vi "Numeric Output Item Init.vi"(7 "Project In":refnum<class "Project.lvclass">, 8 "error in (no error)":errorcluster, 9 "Numeric UI Elements":T1, 10 "Output":T2, 11 "VI in":refnum<vi>) -> (0 "error out":errorcluster)   [LabVIEW 2015, in "OutputUI.lvclass"]
uses:
  OutputUI.lvclass
  Step/STEP_OUTPUT.ctl
  Step/OUTPUT_DATA_TYPE.ctl
  OUTPUT_CHECK_TYPE.ctl
  Step/OUTPUT_VALUE_TYPE.ctl
  Project.lvclass
  Step.lvclass
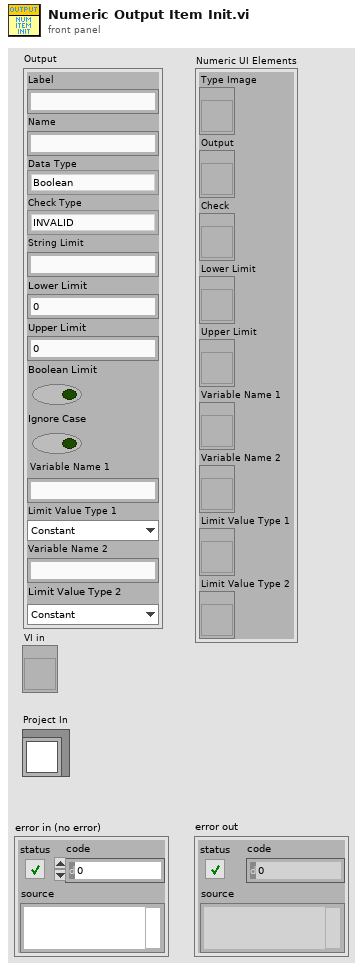
[diagram p1: front panel]
types:
  T1 = cluster{"Type Image":refnum<vi>, "Output":refnum<vi>, "Check":refnum<vi>, "Lower Limit":refnum<vi>, "Upper Limit":refnum<vi>, "Variable Name 1":refnum<vi>, "Variable Name 2":refnum<vi>, "Limit Value Type 1":refnum<vi>, "Limit Value Type 2":refnum<vi>}
  T2 = typedef "Step.lvclass/STEP_OUTPUT.ctl" = cluster{"Label":string, "Name":string, "Data Type":T3, "Check Type":T4, "String Limit":string, "Lower Limit":dbl, "Upper Limit":dbl, "Boolean Limit":bool, "Ignore Case":bool, "Variable Name 1":string, "Limit Value Type 1":T5, "Variable Name 2":string, "Limit Value Type 2":T5}
  T3 = typedef "Step.lvclass/OUTPUT_DATA_TYPE.ctl" = enum16{"Boolean", "String", "Numeric", "Other"}
  T4 = typedef "Step.lvclass/OUTPUT_CHECK_TYPE.ctl" = enum16{"INVALID", "DO_NOT_CHECK", "RECORD", "VARIABLE", "EQUAL", "NOT_EQUAL", "STR_CONTAINS", "STR_START_WITH", "STR_END_WITH", "STR_REGEX_MATCH", "NUM_GT", "NUM_LT", "NUM_GE", "NUM_LE", "NUM_RANGE", "NUM_RANGE_BDY"}
  T5 = typedef "Step.lvclass/OUTPUT_VALUE_TYPE.ctl" = enum16{"Constant", "Variable"}
  T6 = cluster{"Type Image":refnum<vi>, "Output":refnum<vi>, "Check":refnum<vi>}
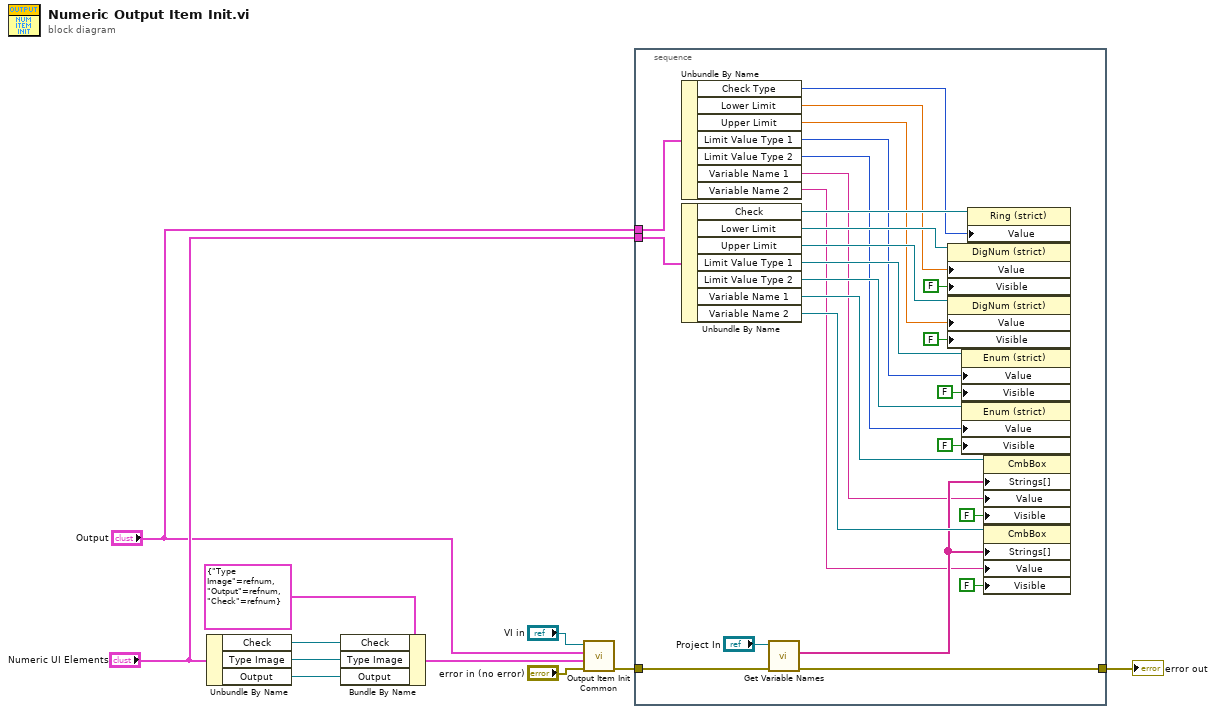
[diagram p0: block diagram]
diagram:
  n1 = Unbundle By Name("Numeric UI Elements") -> ("Check"=w8:refnum<vi>, "Type Image"=w7:refnum<vi>, "Output"=w6:refnum<vi>)
  n2 = Bundle By Name(cluster=T6 {"Type Image"=refnum, "Output"=refnum, "Check"=refnum} ("UI Elements"), "Check"=w8, "Type Image"=w7, "Output"=w6) -> (w5:T6)
  n3 = call "Output Item Init Common.vi"("error in (no error)"="error in (no error)", "UI Elements"=w5, "Output"="Output", "VI in"="VI in") -> ("error out"=w1:errorcluster)  [unwired: 7 in]
  n4 = stacked-sequence {
    tunnel: "Output" -> [w37]
    tunnel: "Numeric UI Elements" -> [w36]
    tunnel: w1 -> [w19]
    tunnel: [w18] -> w11
    frame #0 {
      n5 = Unbundle By Name(w37) -> ("Check Type"=w34:T4, "Lower Limit"=w32:dbl, "Upper Limit"=w30:dbl, "Limit Value Type 1"=w28:T5, "Limit Value Type 2"=w26:T5, "Variable Name 1"=w21:string, "Variable Name 2"=w20:string)
      n6 = Unbundle By Name(w36) -> ("Check"=w35:refnum<vi>, "Lower Limit"=w33:refnum<vi>, "Upper Limit"=w31:refnum<vi>, "Limit Value Type 1"=w29:refnum<vi>, "Limit Value Type 2"=w27:refnum<vi>, "Variable Name 1"=w22:refnum<vi>, "Variable Name 2"=w24:refnum<vi>)
      n7 = call "Get Variable Names.vi"("error in (no error)"=w19, "Project in"="Project In") -> ("error out"=w18:errorcluster, "Variable Names"=w23:string[])  [unwired: 7 in, 1 out]
      n8 = property class="DigNum (strict)"(reference=w33, "Value"=w32, "Visible"=FALSE) -> ()  [unwired: 1 in, 2 out]
      n9 = property class="DigNum (strict)"(reference=w31, "Value"=w30, "Visible"=FALSE) -> ()  [unwired: 1 in, 2 out]
      n10 = property class="Enum (strict)"(reference=w29, "Value"=w28, "Visible"=FALSE) -> ()  [unwired: 1 in, 2 out]
      n11 = property class="Enum (strict)"(reference=w27, "Value"=w26, "Visible"=FALSE) -> ()  [unwired: 1 in, 2 out]
      n12 = property class="Ring (strict)"(reference=w35, "Value"=w34) -> ()  [unwired: 1 in, 2 out]
      n13 = property class="CmbBox"(reference=w22, "Strings[]"=w23, "Value"=w21, "Visible"=FALSE) -> ()  [unwired: 1 in, 2 out]
      n14 = property class="CmbBox"(reference=w24, "Strings[]"=w23, "Value"=w20, "Visible"=FALSE) -> ()  [unwired: 1 in, 2 out]
    }
  }
  "error out" <- w11
